vi "Append Name to Signals.vi"(8 "error in (no error)":errorcluster, 11 "GripsMaster in":refnum<class "GripsMaster.lvclass">) -> (0 "error out":errorcluster, 3 "GripsMaster out":refnum<class "GripsMaster.lvclass">)   [LabVIEW 2011, in "GripsMaster.lvclass"]
uses:
  GripsMaster.lvclass
  GripsMaster.lvclass/GripsMaster.ctl
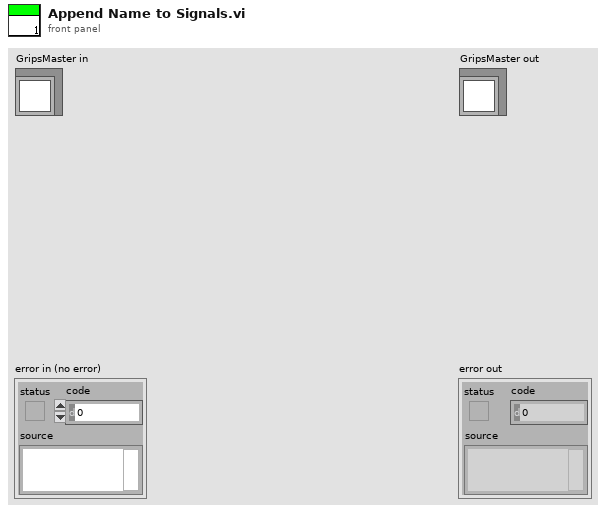
[diagram p1: front panel]
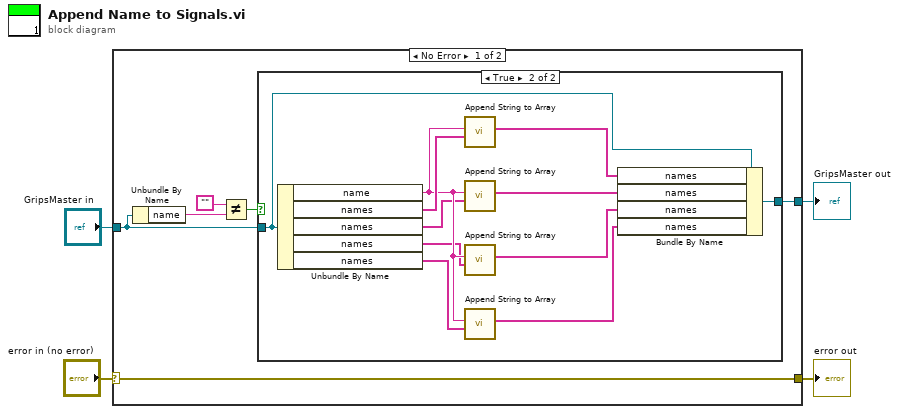
[diagram p0: block diagram]
diagram:
  n1 = case shown="No Error" "error in (no error)" {
    selector: "error in (no error)" -> [w10 w24]
    tunnel: [w10 w24] -> w3
    tunnel: [w5 w23] -> w1
    tunnel: "GripsMaster in" -> [w9 w23]
    frame No Error {
      n2 = Unbundle By Name(w9) -> ("name"=w6:string)
      n3 = Not Equal?(x="", y=w6) -> (x != y?=w8:bool)
      n4 = case shown="True" w8 {
        tunnel: w9 -> [w11 w22]
        tunnel: [w11 w21] -> w5
        frame False {
        }
        frame True {
          n5 = Unbundle By Name(w22) -> ("name"=w15:string, "names"=w20:string[], "names"=w12:string[], "names"=w13:string[], "names"=w14:string[])
          n6 = call "Append String to Array.vi"("array"=w20, "name"=w15) -> ("result"=w19:string[])  [unwired: 9 in]
          n7 = call "Append String to Array.vi"("array"=w12, "name"=w15) -> ("result"=w18:string[])  [unwired: 9 in]
          n8 = call "Append String to Array.vi"("array"=w13, "name"=w15) -> ("result"=w17:string[])  [unwired: 9 in]
          n9 = call "Append String to Array.vi"("array"=w14, "name"=w15) -> ("result"=w16:string[])  [unwired: 9 in]
          n10 = Bundle By Name(cluster=w22, "names"=w19, "names"=w18, "names"=w17, "names"=w16) -> (w21:refnum<class "GripsMaster.lvclass">)
        }
      }
    }
    frame Error {
    }
  }
  "error out" <- w3
  "GripsMaster out" <- w1
